vi "Read Attributes.vi"(11 "Return Devices to Load IDs Msg":refnum<class "Return Devices to Load IDs Msg.lvclass">) -> (2 "Payload":cluster{"Device IDs":T1[], "Microgrid ID":u8}={"Device IDs"=[], "Microgrid ID"=1} {"Microgrid ID" min=1 max=232 step=1})   [LabVIEW 2018, in "Devices to Load Config Actor.lvlib" / "Return Devices to Load IDs Msg.lvclass"]
uses:
  Return Devices to Load IDs Msg.lvclass
  <vilib>/ORNL/CSEISMIC DDS/CSEISMIC DDS Base/Data Types/Controls/DeviceID.ctl
  Return Devices to Load IDs Msg.lvclass/Return Devices to Load IDs Msg.ctl
  <vilib>/ORNL/CSEISMIC DDS/CSEISMIC DDS Base/CSEISMIC DDS.lvclass
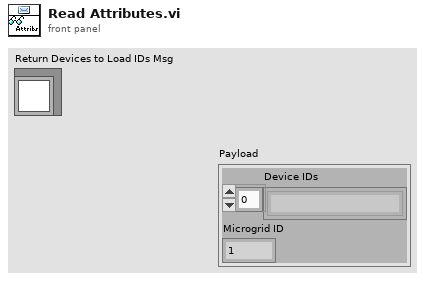
[diagram p1: front panel]
types:
  T1 = typedef "CSEISMIC DDS.lvlib/CSEISMIC DDS.lvclass/DeviceID.ctl" = string
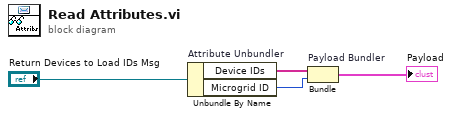
[diagram p0: block diagram]
diagram:
  n1 = Unbundle By Name "Attribute Unbundler"("Return Devices to Load IDs Msg") -> ("Device IDs"=w2:T1[], "Microgrid ID"=w1:u8)
  n2 = Bundle "Payload Bundler"("Device IDs"=w2, "Microgrid ID"=w1) -> (→"Payload":cluster{"Device IDs":T1[], "Microgrid ID":u8})  [unwired: 1 in]
